vi "GetParam.vi"(8 "error in (no error)":errorcluster caption="entrée d'erreur (pas d'erreur)", 11 "binarize.lvclass":refnum<class "binarize.lvclass">) -> (0 "error out":errorcluster caption="sortie d'erreur", 2 "binarize":cluster{"threshold":dbl, "copy":bool}={"threshold"=0.0, "copy"=TRUE}, 3 "binarize.lvclass":refnum<class "binarize.lvclass">)   [LabVIEW 2020, in "binarize.lvclass"]
doc: "Get Parameters"
uses:
  binarize.lvclass
  binarize.lvclass/binarize.ctl
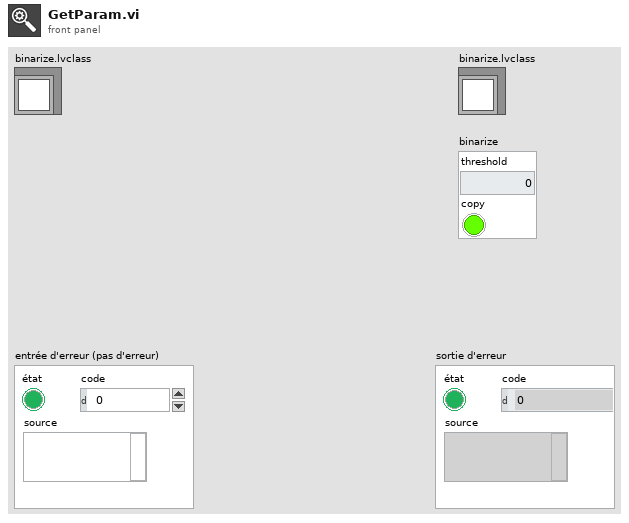
[diagram p1: front panel]
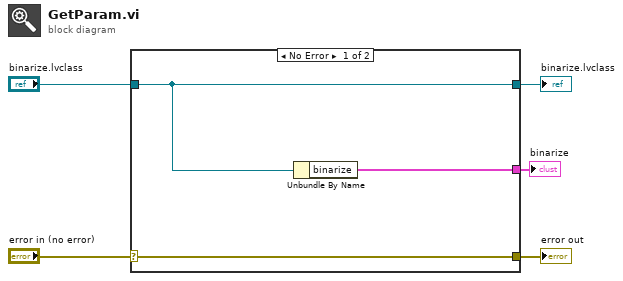
[diagram p0: block diagram]
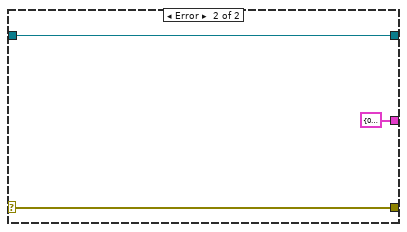
[diagram p2: hidden frame]
diagram:
  n1 = case shown="No Error" "error in (no error)" {
    selector: "error in (no error)" -> [w8 w10]
    tunnel: [w8 w10] -> w4
    tunnel: [w7 w11] -> w2
    tunnel: "binarize.lvclass" -> [w7 w11]
    tunnel: [w6 cluster{"threshold":dbl, "copy":bool} {"threshold"=0.0, "copy"=FALSE} ("binarize")] -> w1
    frame No Error {
      n2 = Unbundle By Name(w7) -> ("binarize"=w6:cluster{"threshold":dbl, "copy":bool})
    }
    frame Error {
    }
  }
  "error out" <- w4
  "binarize.lvclass" <- w2
  "binarize" <- w1
